vi "GetTerms3.vi"(0 "XRef":T15, 1 "State In":T9={"Input Type"=variant(dbl 0.0), "Width"=0, "Typedef Name"="", "Value Type"=variant, "Selection"=0, "Options"=[], "Selections"=[], "Display Selections"=[], "Element Names"=[], "Typedef Name Width"=0, "Display Selection Width"=[], "Code Generated"=FALSE, "Is DVR"=FALSE, "Write Lock"=FALSE}) -> (14 "Terms":T1)   [LabVIEW 2015, in "Read-Write-Signals.xnode"]
doc: "This ability VI is used to describe your terminals to LabVIEW. Terms is an array of clusters describing the XNode's terminals.\n ID: A unique string identifying the terminal.\n Name: The name of the terminal visible to the user. Remember to localize it.\n Type: The data type of the terminal (as a Variant). The data put in the variant will be used as the default for the input terminal if it's left unwired.\n Bounds: A rectangle defining the bounds of the terminal relative to the bounds of the XNode. The bounds must be within the bounds of the XNode, and for whiskers to draw properly, they must be flush with at least one side of the XNode.\n Input?: Indicates whether or not this terminals is an input.\n Required?: Indicates whether the user must wire this terminal for the XNode to not be broken. Ignored on outputs.\n Recommended?: Indicates whether the terminal is recommended.\n Hidden?: Indicates whether the terminal is hidden. When a terminal is hidden, it cannot be wired to via user interaction or scripting. However, if it is already wired to when the hidden flag is changed to true, it will remain wired.\n Adaptive?: Indicates that the term should change to match the type of its source if it is wired.\n Direction?: Indicates what direction the wire stub should point. Choose auto to let LV decide based on the terms bounds being on the nodes edge.\n \n The IDs are used by LabVIEW to keep track of your terminals. When you respecify your terminals, LabVIEW can tell whther terminals are new, deleted, or moved by the unique IDs. The order is irrelevant. If you move a terminal, then any wire connected to it will move with it.\n \n If you want to update your terminals, you should return the UpdateTerms reply in one of your ability VIs.\n\nDefault behavior: None.\n\nThis ability does not provide UI and OS messages are not handled."
uses:
  Read-Write-Signals.xnode
  <vilib>/XNodeSupport/XNodeXNodeRef.ctl
  State.ctl
  Read-Write-Signals Item.ctl
  Read-Write-Signals Sub Item.ctl
  Read-Write-Signals Sub Item Type.ctl
  Read-Write-Signals Selection.ctl
  Read-Write-Signals Display Selection.ctl
  <vilib>/XNodeSupport/XNodeTerm3Array.ctl
  <vilib>/XNodeSupport/XNodeTerm3.ctl
  <vilib>/XNodeSupport/XNodeString.ctl
  <vilib>/XNodeSupport/XNodeVariant.ctl
  <vilib>/XNodeSupport/XNodeRect32.ctl
  <vilib>/XNodeSupport/XNodeInt.ctl
  <vilib>/XNodeSupport/XNodeBool.ctl
  <vilib>/XNodeSupport/XNodeTermDirection.ctl
  <vilib>/XNodeSupport/NI_XNodeSupport.lvlib
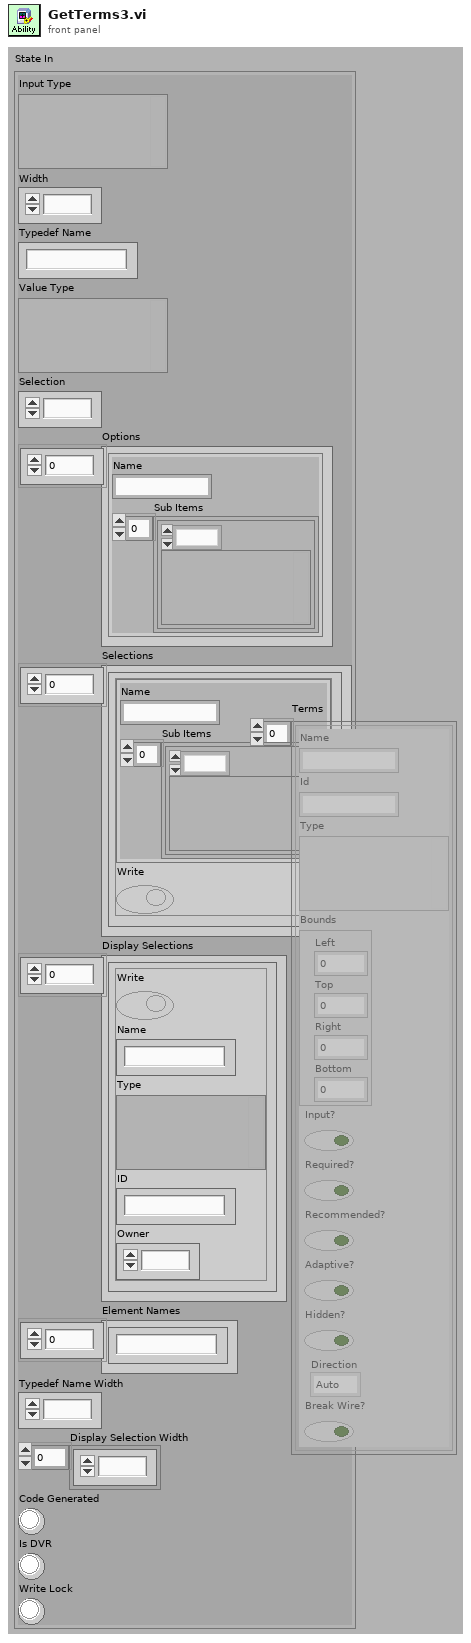
[diagram p1: front panel]
types:
  T1 = typedef "NI_XNodeSupport.lvlib/XNodeTerm3Array.ctl" = T2[]
  T2 = typedef "NI_XNodeSupport.lvlib/XNodeTerm3.ctl" = cluster{"Name":T3, "Id":T3, "Type":T4, "Bounds":T5, "Input?":T7, "Required?":T7, "Recommended?":T7, "Adaptive?":T7, "Hidden?":T7, "Direction":T8, "Break Wire?":T7}
  T3 = typedef "NI_XNodeSupport.lvlib/XNodeString.ctl" = string
  T4 = typedef "NI_XNodeSupport.lvlib/XNodeVariant.ctl" = variant
  T5 = typedef "NI_XNodeSupport.lvlib/XNodeRect32.ctl" = cluster{"Left":T6, "Top":T6, "Right":T6, "Bottom":T6}
  T6 = typedef "NI_XNodeSupport.lvlib/XNodeInt.ctl" = i32
  T7 = typedef "NI_XNodeSupport.lvlib/XNodeBool.ctl" = bool
  T8 = typedef "NI_XNodeSupport.lvlib/XNodeTermDirection.ctl" = enum32{"Auto", "Up", "Down", "Left", "Right", "Center"}
  T9 = typedef "Read-Write-Signals.xnode/State.ctl" = cluster{"Input Type":variant, "Width":i32, "Typedef Name":string, "Value Type":variant, "Selection":i32, "Options":T10[], "Selections":T13[], "Display Selections":T14[], "Element Names":string[], "Typedef Name Width":i32, "Display Selection Width":i32[], "Code Generated":bool, "Is DVR":bool, "Write Lock":bool}
  T10 = typedef "Read-Write-Signals Item.ctl" = cluster{"Name":string, "Sub Items":T11[]}
  T11 = typedef "Read-Write-Signals Sub Item.ctl" = cluster{"Type":T12, "Value":variant}
  T12 = typedef "Read-Write-Signals Sub Item Type.ctl" = enum8{"Cluster Element", "Array Element", "Subarray"}
  T13 = typedef "Read-Write-Signals Selection.ctl" = cluster{"Item":T10, "Write":bool}
  T14 = typedef "Read-Write-Signals Display Selection.ctl" = cluster{"Write":bool, "Name":string, "Type":variant, "ID":string, "Owner":i32}
  T15 = typedef "NI_XNodeSupport.lvlib/XNodeXNodeRef.ctl" = refnum<vi>
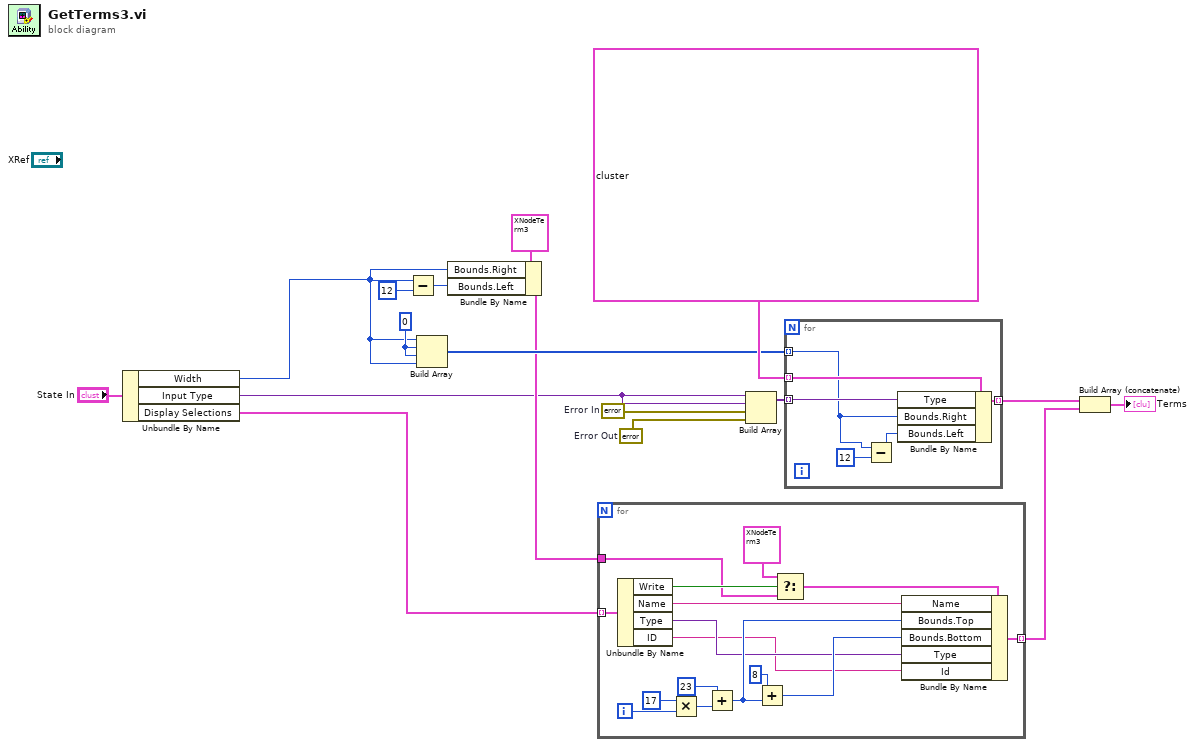
[diagram p0: block diagram]
diagram:
  w10 = 0 ("element")
  w15 = errorcluster {"status"=FALSE, "code"=0, "source"=""}  # Error Out
  w16 = errorcluster {"status"=FALSE, "code"=0, "source"=""}  # Error In
  n1 = Unbundle By Name("State In") -> ("Width"=w1:i32, "Input Type"=w4:variant, "Display Selections"=w3:T14[])
  n2 = Subtract(x=w1, y=12) -> (x-y=w7:i32)
  n3 = Build Array(w1, w10, w10, w1) -> (w9:i32[])
  n4 = Bundle By Name(cluster=T2 {"Name"="", "Id"="", "Type"=variant, "Bounds"={"Left"=86, "Top"=0, "Right"=98, "Bottom"=0}, "Input?"=FALSE, "Required?"=FALSE, "Recommended?"=TRUE, "Adaptive?"=FALSE, "Hidden?"=FALSE, "Direction"=enum."Auto", "Break Wire?"=FALSE} ("Term 3"), "Bounds.Right"=w1, "Bounds.Left"=w7) -> (w6:T2)
  n5 = for {
    tunnel: w3 -> [w33] mode=indexing
    tunnel: [w23] -> w12 mode=indexing
    tunnel: w6 -> [w21]
    i -> [w22]
    n6 = Unbundle By Name(w33) -> ("Write"=w32:bool, "Name"=w20:string, "Type"=w19:variant, "ID"=w18:string)
    n7 = Multiply(x=17, y=w22) -> (x*y=w28:i32)
    n8 = Add(x=23, y=w28) -> (x+y=w25:i32)
    n9 = Add(x=8, y=w25) -> (x+y=w24:i32)
    n10 = Select(t=T2 {"Name"="", "Id"="", "Type"=variant, "Bounds"={"Left"=0, "Top"=0, "Right"=8, "Bottom"=0}, "Input?"=TRUE, "Required?"=TRUE, "Recommended?"=TRUE, "Adaptive?"=FALSE, "Hidden?"=FALSE, "Direction"=enum."Auto", "Break Wire?"=FALSE} ("Term 3"), s=w32, f=w21) -> (s? t:f=w30:T2)
    n11 = Bundle By Name(cluster=w30, "Name"=w20, "Bounds.Top"=w25, "Bounds.Bottom"=w24, "Type"=w19, "Id"=w18) -> (w23:T2)
  }
  n12 = Build Array(w4, w4, w16, w15) -> (w17:variant[])
  n13 = for {
    tunnel: T2[] [{"Name"="Signals Out", "Id"="out", "Type"=variant, "Bounds"={"Left"=86, "Top"=0, "Right"=98, "Bottom"=8}, "Input?"=FALSE, "Required?"=FALSE, "Recommended?"=TRUE, "Adaptive?"=FALSE, "Hidden?"=FALSE, "Direction"=enum."Auto", "Break Wire?"=FALSE}, {"Name"="Signals In", "Id"="in", "Type"=variant, "Bounds"={"Left"=0, "Top"=0, "Right"=8, "Bottom"=8}, "Input?"=TRUE, "Required?"=TRUE, "Recommended?"=TRUE, "Adaptive?"=FALSE, "Hidden?"=FALSE, "Direction"=enum."Auto", "Break Wire?"=FALSE}, {"Name"="Error In", "Id"="ein", "Type"=variant, "Bounds"={"Left"=0, "Top"=10, "Right"=8, "Bottom"=18}, "Input?"=TRUE, "Required?"=FALSE, "Recommended?"=TRUE, "Adaptive?"=FALSE, "Hidden?"=FALSE, "Direction"=enum."Auto", "Break Wire?"=FALSE}, {"Name"="Error Out", "Id"="eout", "Type"=variant, "Bounds"={"Left"=86, "Top"=10, "Right"=98, "Bottom"=18}, "Input?"=FALSE, "Required?"=FALSE, "Recommended?"=TRUE, "Adaptive?"=FALSE, "Hidden?"=FALSE, "Direction"=enum."Auto", "Break Wire?"=FALSE}] -> [w39] mode=indexing
    tunnel: w17 -> [w37] mode=indexing
    tunnel: [w38] -> w13 mode=indexing
    tunnel: w9 -> [w35] mode=indexing
    n14 = Subtract(x=w35, y=12) -> (x-y=w34:i32)
    n15 = Bundle By Name(cluster=w39, "Type"=w37, "Bounds.Right"=w35, "Bounds.Left"=w34) -> (w38:T2)
  }
  n16 = Build Array (concatenate)(w13, w12) -> (→"Terms":T2[])
